vi "数据上传03.vi"(5 "产品ID":string, 6 "油封压入力":dbl, 7 "堵头2压入位移":dbl, 8 "堵头2压入力":dbl, 9 "堵头1压入位移":dbl, 10 "堵头1压入力":dbl, 11 "合格03":bool) -> ()   [LabVIEW 2011]
uses:
  <vilib>/Utility/error.llb/whitespace.ctl
panel:
  in  "error in (no error)":errorcluster
  out "error out":errorcluster
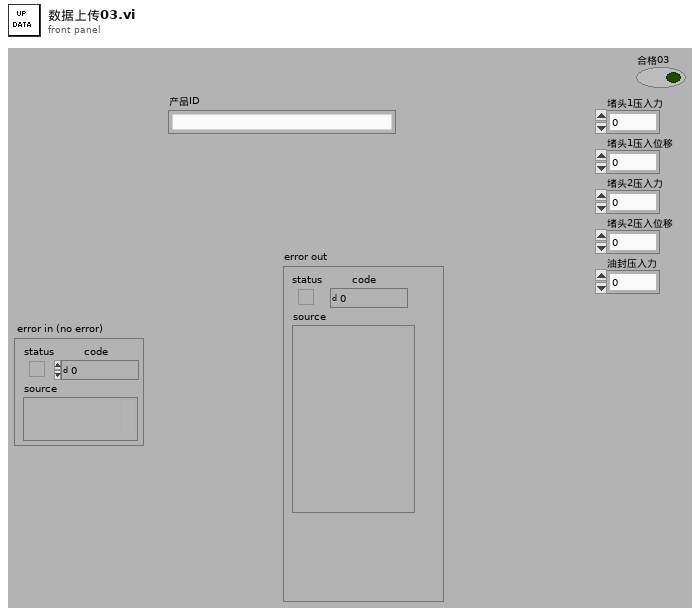
[diagram p1: front panel]
types:
  T1 = typedef "whitespace.ctl" = u16
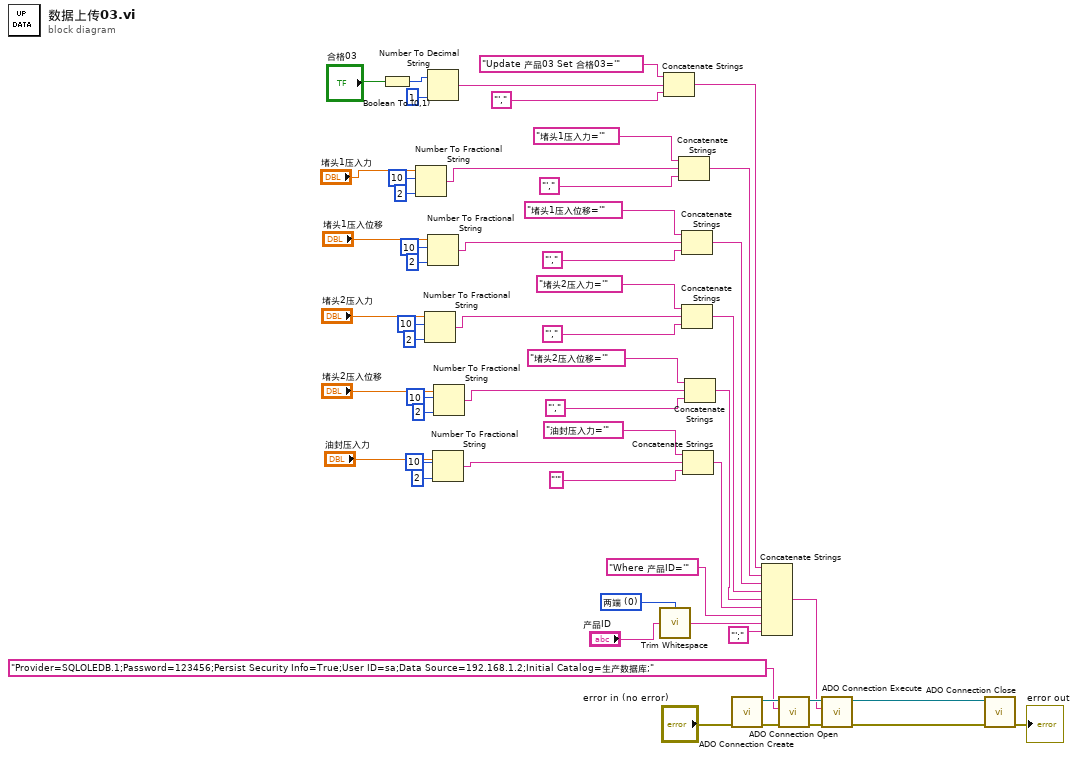
[diagram p0: block diagram]
diagram:
  w49 = T1 0 items=["两端", "字符串首端", "字符串末端"] ("location (both)")
  n1 = Boolean To (0,1)(Boolean="合格03") -> (0, 1=w23:i16)
  n2 = Number To Fractional String(number="堵头1压入力", width (-)=i16 10 ("宽度(-)"), precision (6)=i16 2 ("宽度(-)")) -> (F-format string=w18:string)  [unwired: 1 in]
  n3 = Number To Fractional String(number="堵头2压入力", width (-)=i16 10 ("宽度(-)"), precision (6)=i16 2 ("宽度(-)")) -> (F-format string=w10:string)  [unwired: 1 in]
  n4 = Number To Decimal String(number=w23, width (-)=i16 1 ("宽度(-)")) -> (decimal integer string=w21:string)
  n5 = Number To Fractional String(number="堵头1压入位移", width (-)=i16 10 ("宽度(-)"), precision (6)=i16 2 ("宽度(-)")) -> (F-format string=w12:string)  [unwired: 1 in]
  n6 = Number To Fractional String(number="油封压入力", width (-)=i16 10 ("宽度(-)"), precision (6)=i16 2 ("宽度(-)")) -> (F-format string=w6:string)  [unwired: 1 in]
  n7 = Number To Fractional String(number="堵头2压入位移", width (-)=i16 10 ("宽度(-)"), precision (6)=i16 2 ("宽度(-)")) -> (F-format string=w8:string)  [unwired: 1 in]
  n8 = call <vilib>:"Trim Whitespace.vi"("string"="产品ID", "location (both)"=w49) -> ("trimmed string"=w47:string)
  n9 = Concatenate Strings("Update 产品03 Set 合格03='" ("字符串"), w21, "'," ("字符串")) -> (w30:string)
  n10 = Concatenate Strings("堵头1压入力='" ("字符串"), w18, "'," ("字符串")) -> (w29:string)
  n11 = Concatenate Strings("堵头1压入位移='" ("字符串"), w12, "'," ("字符串")) -> (w28:string)
  n12 = Concatenate Strings("堵头2压入力='" ("字符串"), w10, "'," ("字符串")) -> (w27:string)
  n13 = Concatenate Strings("油封压入力='" ("字符串"), w6, "'" ("字符串")) -> (w25:string)
  n14 = Concatenate Strings("堵头2压入位移='" ("字符串"), w8, "'," ("字符串")) -> (w26:string)
  n15 = call "ADO Connection Create.vi"("error in (no error)"="error in (no error)") -> ("error out"=w56:errorcluster, "ADODB._Connection Out"=w57:refnum<k7>)  [unwired: 9 out]
  n16 = Concatenate Strings(w30, w29, w28, w27, w26, w25, "Where 产品ID='" ("字符串"), w47, "';" ("字符串")) -> (w45:string)
  n17 = call "ADO Connection Open.vi"("error in (no error)"=w56, "ConnectionString"="Provider=SQLOLEDB.1;Password=123456;Persist Security Info=True;User ID=sa;Data Source=192.168.1.2;Initial Catalog=生产数据库;" ("字符串 2"), "ADODB._Connection In"=w57) -> ("error out"=w55:errorcluster, "ADODB._Connection Out"=w54:refnum<k7>)  [unwired: 7 out]
  n18 = call "ADO Connection Execute.vi"("error in (no error)"=w55, "CommandText"=w45, "ADODB._Connection In"=w54) -> ("error out"=w44:errorcluster, "ADODB._Connection Out"=w52:refnum<k7>)  [unwired: 7 out]
  n19 = call "ADO Connection Close.vi"("error in (no error)"=w44, "ADODB._Connection In"=w52) -> ("error out"=→"error out":errorcluster)  [unwired: 9 out]
